vi "Vacuum Switch Panel.vi"() -> ()   [LabVIEW 2018]
uses:
  Classes/Controller/Controller.lvclass
  Classes/Controller/I-O/I-O.lvclass
panel:
  in  "Turn off all":bool
  out "error out":errorcluster
  out "Compression Sensor":bool
  out "Sensor Channel":dbl=6.0
  out "Sensor":bool
  out "sensor pin number":i32=3
  out "tray sensor":bool
  out "secondary valve sensor":bool
  out "primary valve sensor":bool
  in  "Turn on secondary vacuum":bool
  in  "turn on primary vacuum":bool
  in  "secure tray":bool
  out "Valve Channel":dbl=6.0
  in  "Type":enum16{"O ring Vac", "Baseplate Vac"}(ring)
  in  "Position":i32=1 min=1 max=2
  in  "Region":i32=1 min=1 max=2
  in  "On/Off":bool
  in  "Stop":bool
  in  "error in (no error)":errorcluster
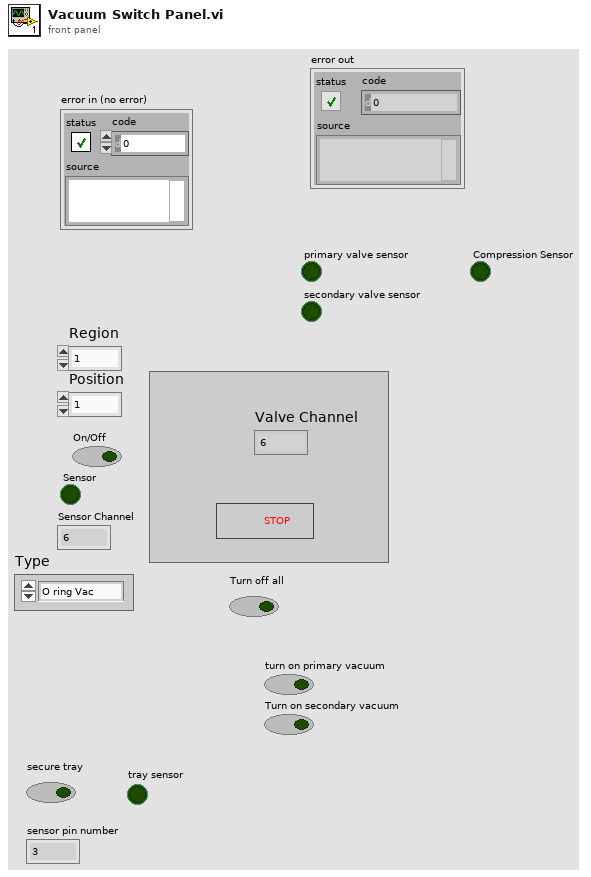
[diagram p1: front panel]
types:
  T1 = typedef "Controller.lvclass/Controllers.ctl" = cluster{"I-O.lvclass":refnum<class "I-O.lvclass">, "Gantry":refnum<k24>, "Dispenser":refnum<visa-resource-name>}
  T2 = typedef "I-O.lvclass/Pin Map.ctl" = cluster{"Region Valves":i32[], "Extra Valves":dbl[][][], "Tool Primary Valve":i32, "Tool Secondary Valve":i32, "Region Sensors":i32[], "Extra Sensors":dbl[][][], "Tool Primary Sensor":dbl, "Tool Secondary Sensor":dbl, "Compression Sensor":dbl, "5V":i32, "Dispenser Sensor":dbl}
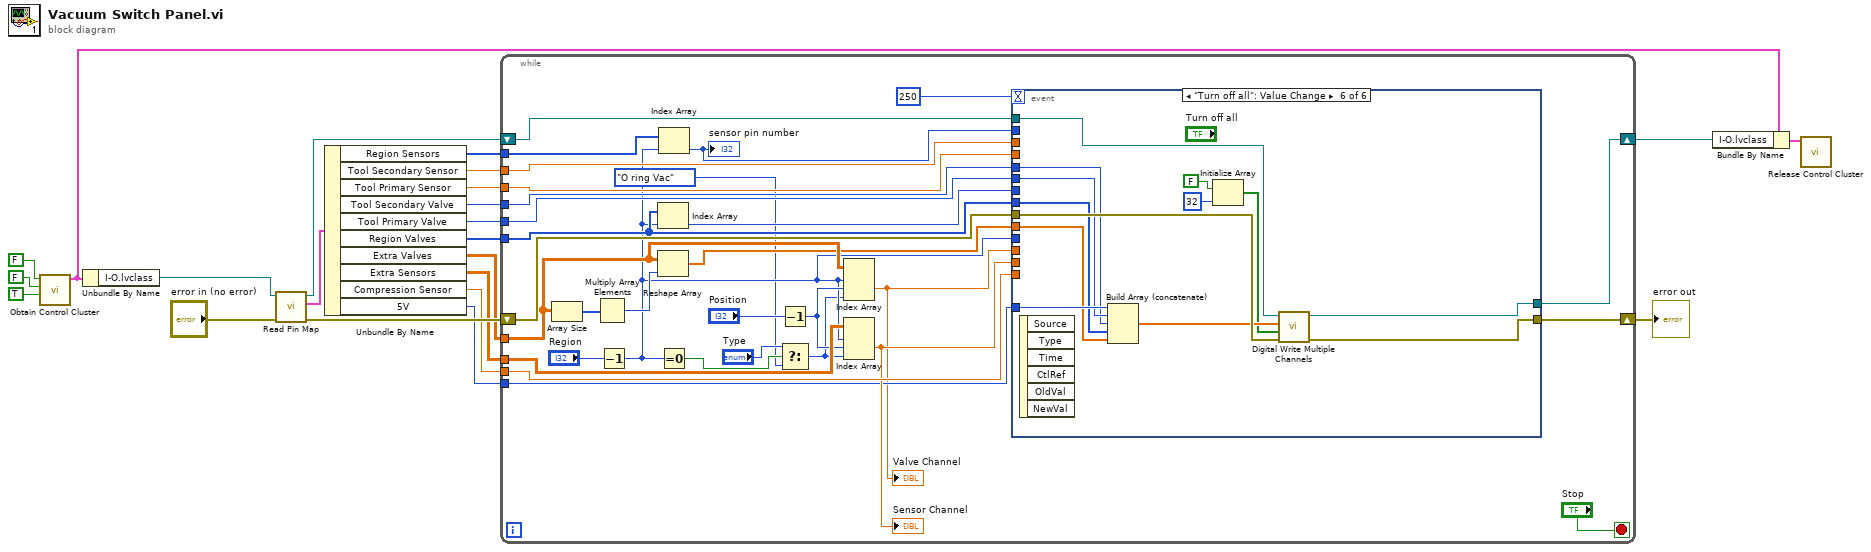
[diagram p0: block diagram]
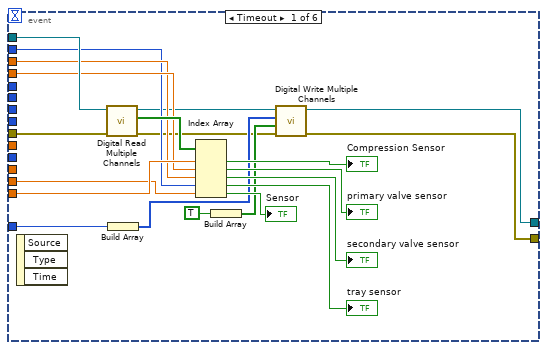
[diagram p2: hidden frame]
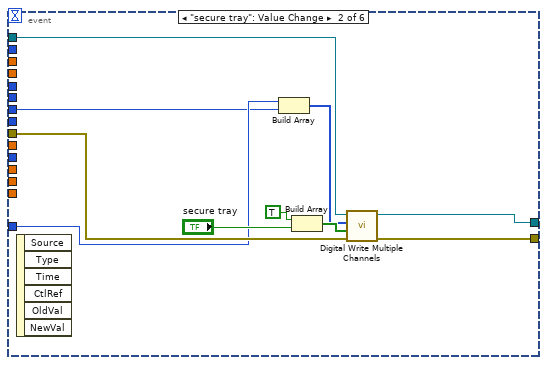
[diagram p3: hidden frame]
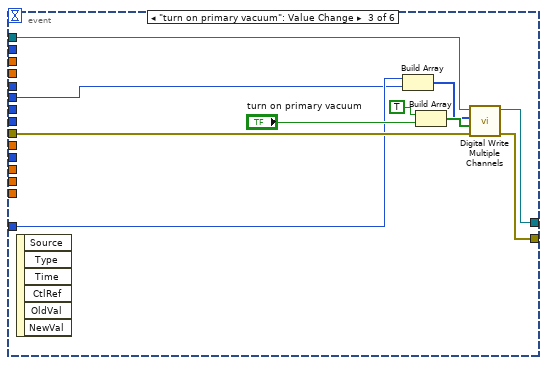
[diagram p4: hidden frame]
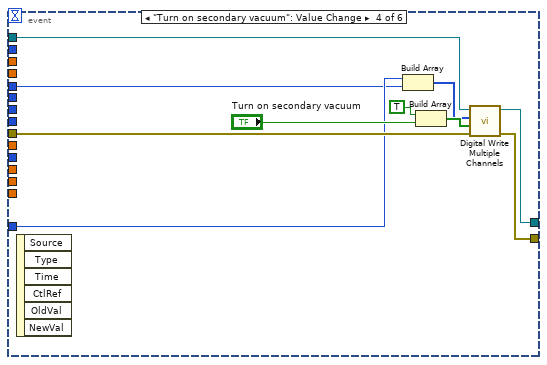
[diagram p5: hidden frame]
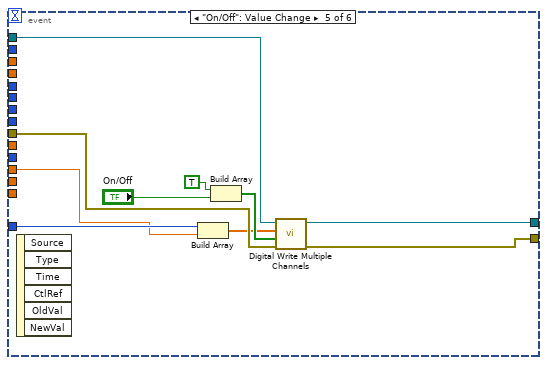
[diagram p6: hidden frame]
diagram:
  n1 = call "Obtain Control Cluster.vi"("I/O"=TRUE, "Dispense"=FALSE, "Motion"=FALSE) -> ("Control Out"=w4:T1)  [unwired: 8 in]
  n2 = Unbundle By Name(w4) -> ("I-O.lvclass"=w18:refnum<class "I-O.lvclass">)
  n3 = call-dynamic "Read Pin Map.vi"("error in (no error)"="error in (no error)", "I-O in"=w18) -> ("error out"=w16:errorcluster, "Pin Map 2"=w22:T2, "I-O out"=w15:refnum<class "I-O.lvclass">)  [unwired: 7 in]
  n4 = Unbundle By Name(w22) -> ("Region Sensors"=w11:i32[], "Tool Secondary Sensor"=w12:dbl, "Tool Primary Sensor"=w13:dbl, "Tool Secondary Valve"=w7:i32, "Tool Primary Valve"=w8:i32, "Region Valves"=w5:i32[], "Extra Valves"=w6:dbl[][][], "Extra Sensors"=w10:dbl[][][], "Compression Sensor"=w14:dbl, "5V"=w9:i32)
  n5 = while {
    shift-right: [w50] -> w2
    shift-left: w15 -> [w51]
    shift-right: [w49] -> w1
    shift-left: w16 -> [w52]
    tunnel: w11 -> [w46]
    tunnel: w14 -> [w45]
    tunnel: w13 -> [w44]
    tunnel: w12 -> [w43]
    tunnel: w10 -> [w42]
    tunnel: w9 -> [w39]
    tunnel: w8 -> [w38]
    tunnel: w7 -> [w37]
    tunnel: w6 -> [w31]
    tunnel: w5 -> [w33]
    stop <- "Stop" stop-if-true
    n6 = Array Size(array=w31) -> (size(s)=w32:i32[])
    n7 = Multiply Array Elements(1:w32) -> (0:w30:i32)
    n8 = Decrement(x="Region") -> (x-1=w27:i32)
    n9 = Index Array(array=w33, index=w27) -> (element=w34:i32)
    n10 = Reshape Array(w31, w30) -> (w29:dbl[])
    n11 = Index Array(array=w46, index=w27) -> (element=w41:i32)
    "sensor pin number" <- w41
    n12 = Equal To 0?(x=w27) -> (x = 0?=w26:bool)
    n13 = Decrement(x="Position") -> (x-1=w36:i32)
    n14 = Select(t="Type", s=w26, f=enum16{"O ring Vac", "Baseplate Vac"}."O ring Vac") -> (s? t:f=w24:enum16{"O ring Vac", "Baseplate Vac"})
    n15 = Index Array(array=w31, index (dim 0)=w27, index (dim 1)=w36, index (dim 2)=w24) -> (element=w35:dbl)
    "Valve Channel" <- w35
    n16 = Index Array(array=w42, index (dim 0)=w27, index (dim 1)=w36, index (dim 2)=w24) -> (element=w40:dbl)
    "Sensor Channel" <- w40
    n17 = event shown="[5] \"Turn off all\": Value Change" {
      selector: _ -> [_ _ _ _ _ _]
      dyn-events: _ -> [_ _ _ _ _ _]
      timeout: 250 -> [_ _ _ _ _ _]
      tunnel: w52 -> [w74 w81 w90 w102 w109 w124]
      tunnel: w51 -> [w73 w84 w94 w101 w112 w127]
      tunnel: [w60 w83 w93 w100 w111 w126] -> w50
      tunnel: [w54 w82 w89 w99 w110 w125] -> w49
      tunnel: w27 -> [_ _ _ _ _ _]
      tunnel: w45 -> [w66 _ _ _ _ _]
      tunnel: w44 -> [w65 _ _ _ _ _]
      tunnel: w43 -> [w64 _ _ _ _ _]
      tunnel: w40 -> [w63 _ _ _ _ _]
      tunnel: w41 -> [w62 _ _ _ _ _]
      tunnel: w39 -> [w58 w76 w87 w97 w107 w123]
      tunnel: w38 -> [_ _ w86 _ _ w122]
      tunnel: w37 -> [_ _ _ w96 _ w121]
      tunnel: w35 -> [_ _ _ _ w105 _]
      tunnel: w34 -> [_ w75 _ _ _ _]
      tunnel: w33 -> [_ _ _ _ _ w120]
      tunnel: w29 -> [_ _ _ _ _ w119]
      event Timeout {
        n18 = event-data() -> ()  [unwired: 1 in, 3 out]
        n19 = call-dynamic "Digital Read Multiple Channels.vi"("error in (no error)"=w74, "I-O in"=w73) -> ("error out"=w55:errorcluster, "Array 2"=w72:bool[], "I-O out"=w61:refnum<class "I-O.lvclass">)  [unwired: 7 in]
        n20 = Build Array(w58) -> (w59:i32[])
        n21 = Index Array(array=w72, index #1=w66, index #2=w65, index #3=w64, index #4=w62, index #5=w63) -> (element #1=→"Compression Sensor":bool, element #2=→"primary valve sensor":bool, element #3=→"secondary valve sensor":bool, element #4=→"tray sensor":bool, element #5=→"Sensor":bool)
        n22 = Build Array(TRUE) -> (w57:bool[])
        n23 = call-dynamic "Digital Write Multiple Channels.vi"("error in (no error)"=w55, "values"=w57, "indices"=w59, "I-O in"=w61) -> ("error out"=w54:errorcluster, "I-O out"=w60:refnum<class "I-O.lvclass">)  [unwired: 6 in]
      }
      event "secure tray": Value Change {
        n24 = event-data() -> ()  [unwired: 1 in, 6 out]
        n25 = Build Array(w76, w75) -> (w78:i32[])
        n26 = Build Array(TRUE ("element"), "secure tray") -> (w79:bool[])
        n27 = call-dynamic "Digital Write Multiple Channels.vi"("error in (no error)"=w81, "values"=w79, "indices"=w78, "I-O in"=w84) -> ("error out"=w82:errorcluster, "I-O out"=w83:refnum<class "I-O.lvclass">)  [unwired: 6 in]
      }
      event "turn on primary vacuum": Value Change {
        n28 = event-data() -> ()  [unwired: 1 in, 6 out]
        n29 = Build Array(w87, w86) -> (w85:i32[])
        n30 = Build Array(TRUE ("element"), "turn on primary vacuum") -> (w91:bool[])
        n31 = call-dynamic "Digital Write Multiple Channels.vi"("error in (no error)"=w90, "values"=w91, "indices"=w85, "I-O in"=w94) -> ("error out"=w89:errorcluster, "I-O out"=w93:refnum<class "I-O.lvclass">)  [unwired: 6 in]
      }
      event "Turn on secondary vacuum": Value Change {
        n32 = event-data() -> ()  [unwired: 1 in, 6 out]
        n33 = Build Array(w97, w96) -> (w95:i32[])
        n34 = Build Array(TRUE ("element"), "Turn on secondary vacuum") -> (w104:bool[])
        n35 = call-dynamic "Digital Write Multiple Channels.vi"("error in (no error)"=w102, "values"=w104, "indices"=w95, "I-O in"=w101) -> ("error out"=w99:errorcluster, "I-O out"=w100:refnum<class "I-O.lvclass">)  [unwired: 6 in]
      }
      event "On/Off": Value Change {
        n36 = event-data() -> ()  [unwired: 1 in, 6 out]
        n37 = Build Array(w107, w105) -> (w106:dbl[])
        n38 = Build Array(TRUE ("element"), "On/Off") -> (w114:bool[])
        n39 = call-dynamic "Digital Write Multiple Channels.vi"("error in (no error)"=w109, "values"=w114, "indices"=w106, "I-O in"=w112) -> ("error out"=w110:errorcluster, "I-O out"=w111:refnum<class "I-O.lvclass">)  [unwired: 6 in]
      }
      event "Turn off all": Value Change {
        n40 = event-data() -> ()  [unwired: 1 in, 6 out]
        n41 = Build Array (concatenate)(w123, w122, w121, w120, w119) -> (w118:dbl[])
        n42 = Initialize Array(FALSE, 32 ("dimension size")) -> (w115:bool[])
        n43 = call-dynamic "Digital Write Multiple Channels.vi"("error in (no error)"=w124, "values"=w115, "indices"=w118, "I-O in"=w127) -> ("error out"=w125:errorcluster, "I-O out"=w126:refnum<class "I-O.lvclass">)  [unwired: 6 in]
      }
    }
  }
  "error out" <- w1
  n44 = Bundle By Name(cluster=w4, "I-O.lvclass"=w2) -> (w3:T1)
  n45 = call "Release Control Cluster.vi"("output cluster"=w3) -> ()  [unwired: 11 in]
